vi "Get_Driver.vi"(0 "路径":path, 11 "error in (no error)":errorcluster caption="错误输入（无错误）") -> (4 "路径 2":path, 6 "数组":string[](array[string]), 8 "fixture_Driver":string[](array[string]), 10 "Hi-pot_Driver":string[](array[string]), 15 "error out":errorcluster caption="错误输出")   [LabVIEW 2018]
uses:
  <vilib>/Utility/config.llb/Read Key (String).vi
  <vilib>/Utility/config.llb/NI_LVConfig.lvlib
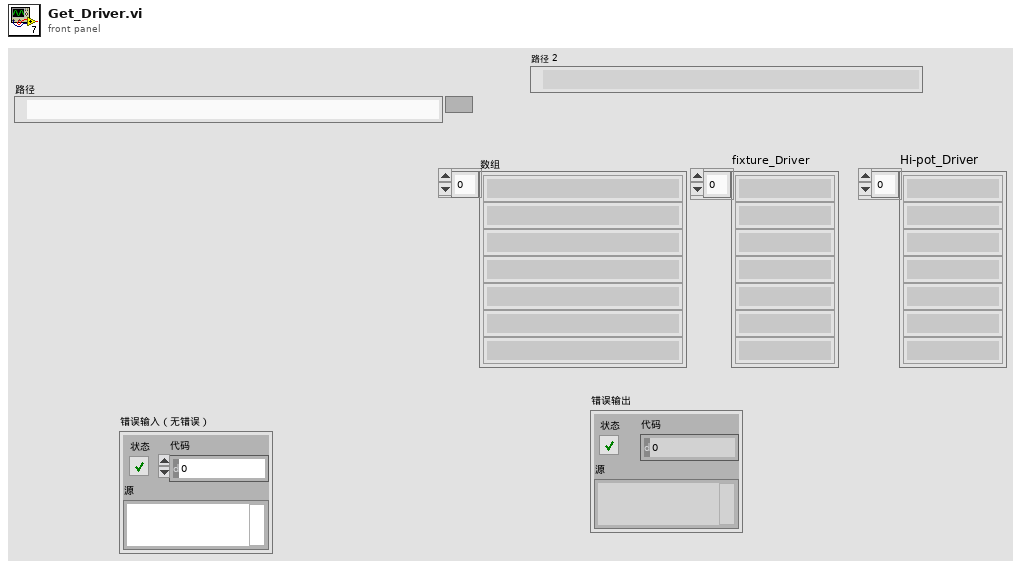
[diagram p1: front panel]
types:
  T1 = typedef "NI_LVConfig.lvlib/Config Data RefNum.ctl" = refnum<k1>
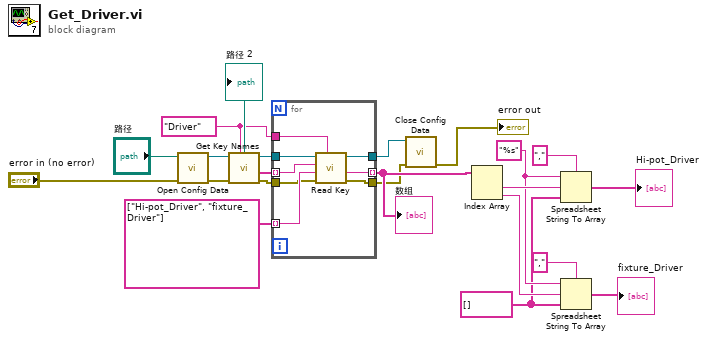
[diagram p0: block diagram]
diagram:
  w10 = "%s"
  w8 = string[] []
  w13 = "Driver" ("section")
  n1 = call <vilib>:"Open Config Data.vi"("error in (no error)"="error in (no error)", "configuration file path"="路径") -> ("error out"=w17:errorcluster, "refnum"=w16:T1)  [unwired: 7 in, 1 out]
  n2 = call <vilib>:"Get Key Names.vi"("section"=w13, "error in (no error)"=w17, "refnum"=w16) -> ("error out"=w5:errorcluster, "key names"=w18:string[], "refnum out"=w19:T1)  [unwired: 5 in, 1 out]
  n3 = for {
    tunnel: w18 -> [w28] mode=indexing
    tunnel: w19 -> [w29]
    tunnel: [w27] -> w21 mode=indexing
    tunnel: [w26] -> w20
    tunnel: string[] ["Hi-pot_Driver", "fixture_Driver"] -> [w25] mode=indexing
    tunnel: w13 -> [w24]
    tunnel: [w23] -> w6
    tunnel: w5 -> [w22]
    n4 = call-poly <vilib>:"Read Key.vi"("section"=w24, "error in (no error)"=w22, "default value"=w25, "key"=w28, "refnum"=w29) -> ("error out"=w23:errorcluster, "value"=w27:string, "refnum out"=w26:T1)  [unwired: 3 in, 1 out]
  }
  "数组" <- w21
  n5 = call <vilib>:"Close Config Data.vi"("error in (no error)"=w6, "refnum"=w20) -> ("error out"=→"error out":errorcluster)  [unwired: 8 in, 1 out]
  n6 = Index Array(array=w21) -> (element #1=w11:string, element #2=w9:string)  [unwired: 2 in]
  n7 = Spreadsheet String To Array(delimiter (Tab)="," ("分隔符(Tab)"), format string=w10, spreadsheet string=w11, array type (2D Dbl)=w8) -> (array=→"Hi-pot_Driver":string[])
  n8 = Spreadsheet String To Array(delimiter (Tab)="," ("分隔符(Tab)"), format string=w10, spreadsheet string=w9, array type (2D Dbl)=w8) -> (array=→"fixture_Driver":string[])
  "路径 2" <- "路径"
